vi "Get AI historian from PGserver v1.vi"(4 "time":timestamp, 8 "error in":errorcluster, 9 "ParamColumns":string[](array[string])=["EPBP1_XQ01", "EPBP2_XQ01", "EPBP3_XQ01"], 10 "ParamTable":string="EP_XQ.1802", 11 "conn":u32) -> (0 "error out":errorcluster, 3 "Out":cluster{"time stamp":timestamp, dbl[]}[](array[cluster]))   [LabVIEW 2019, in "Inputs.lvlib"]
uses:
  Inputs.lvlib
  Database/PostgreSQL2LabVIEW/libpqUtility/libpqutility.lvlib
  Database/PostgreSQL.lvlib
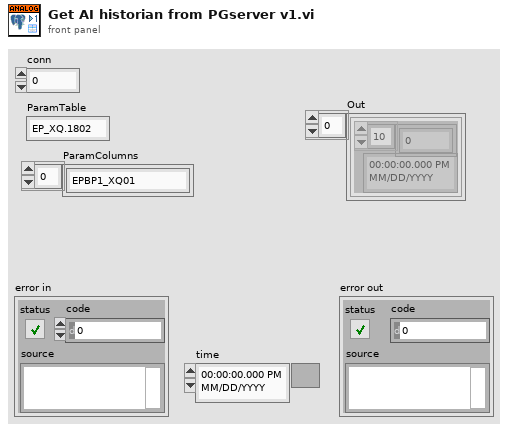
[diagram p1: front panel]
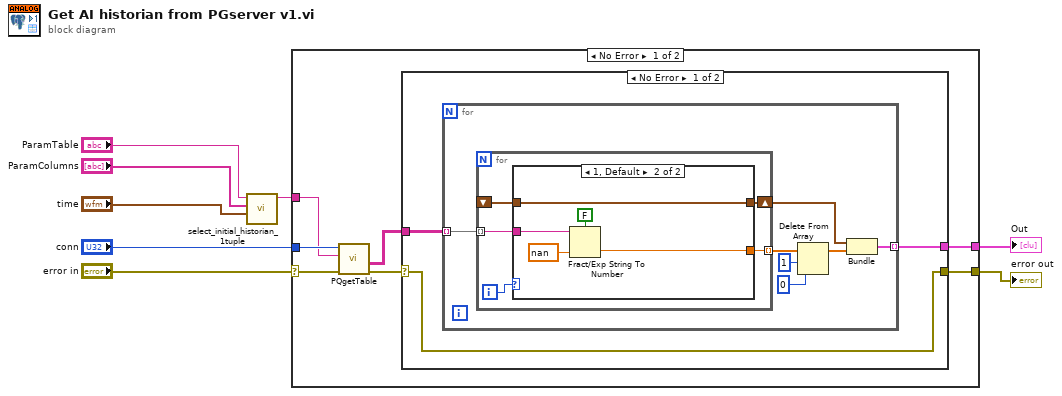
[diagram p0: block diagram]
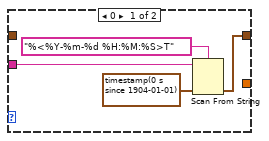
[diagram p2: hidden frame]
diagram:
  n1 = call "select_initial_historian_1tuple.vi"("time"="time", "Column table"="ParamColumns", "table"="ParamTable") -> ("parameters"=w4:string)  [unwired: 8 in]
  n2 = case shown="No Error" "error in" {
    selector: "error in" -> [w14 w41]
    tunnel: "conn" -> [w15 _]
    tunnel: w4 -> [w13 _]
    tunnel: [w9 w41] -> w6
    tunnel: [w11 _] -> w1
    frame No Error {
      n3 = call "PQgetTable.vi"("error in"=w14, "query"=w13, "conn"=w15) -> ("error out"=w10:errorcluster, "Data"=w12:string[][])  [unwired: 4 in, 3 out]
      n4 = case shown="No Error" w10 {
        selector: w10 -> [w17 w40]
        tunnel: w12 -> [w18 _]
        tunnel: [w16 _] -> w11
        tunnel: [w17 w40] -> w9
        frame No Error {
          n5 = for {
            tunnel: w18 -> [w25] mode=indexing
            tunnel: [w24] -> w16 mode=indexing
            n6 = for {
              tunnel: w25 -> [w30] mode=indexing
              tunnel: [w29] -> w23 mode=indexing
              shift-right: [w27] -> w22
              shift-left: _ -> [w26]
              i -> [w28]
              n7 = case shown="1, Default" w28 {
                tunnel: w30 -> [w32 w37]
                tunnel: [_ w36] -> w29
                tunnel: [w31 w35] -> w27
                tunnel: w26 -> [_ w35]
                frame 0 {
                  n8 = Scan From String(format string="%<%Y-%m-%d %H:%M:%S>T" ("string"), input string=w32, default 1=timestamp(0 s since 1904-01-01) ("time stamp")) -> (output 1=w31:timestamp)  [unwired: 2 in, 3 out]
                }
                frame 1, Default {
                  n9 = Fract/Exp String To Number(use system decimal point (T)=FALSE, string=w37, default (0 dbl)=nan) -> (number=w36:dbl)  [unwired: 1 in, 1 out]
                }
              }
            }
            n10 = Delete From Array(array=w23, length=1, index=0) -> (array with subset deleted=w20:dbl[])  [unwired: 1 out]
            n11 = Bundle("time stamp"=w22, w20) -> (w24:cluster{"time stamp":timestamp, dbl[]})  [unwired: 1 in]
          }
        }
        frame Error {
        }
      }
    }
    frame Error {
    }
  }
  "Out" <- w1
  "error out" <- w6
